vi "Window-Timelapse editor.vi"() -> ()   [LabVIEW 2013]
uses:
  User Interface/Visualisation/Timelapse Viewer/Typedefs/Custom slider-vertical.ctl
  User Interface/Visualisation/Timelapse Viewer/Typedefs/Timelapse viewer refs.ctl
  User Interface/Visualisation/Timelapse Viewer/Typedefs/Speed Viewer States enum.ctl
  <vilib>/Utility/miscctls.llb/LVPointTypeDef.ctl
  Typedefs/Save-Load enum.ctl
  <vilib>/vision/Image Controls.llb/IMAQ Image.ctl
  User Interface/Visualisation/Functional Imaging Viewer/Typedefs/Get-Set-Clear Control.ctl
  User Interface/Visualisation/Timelapse Viewer/Typedefs/Select Play-Stop button to show.ctl
  <vilib>/Utility/error.llb/DialogType.ctl
  User Interface/Visualisation/Timelapse Viewer/Cam video sync/Typedefs/Cam videos cluster.ctl
  User Interface/Visualisation/Timelapse Viewer/Globals/gl_Time series viewer globals.vi
  Global Variables/General Globals.vi
panel:
  out "Slider at frame #":i32 format="Slider at frame: %.0f"
  in  "Scrollbar":i32(c297)
  in  "Back":bool
  in  "Play":bool
  in  "Stop":bool
  in  "Tab Control":enum32{"Camera videos", "Speed data"}(tab)
  out "Cams":T2 {"Vid4 Rel time (ms)" format="%.0f ms"; "Vid3 Rel time (ms)" format="%.0f ms"; "Vid2 Rel time (ms)" format="%.0f ms"; "Vid1 Rel time (ms)" format="%.0f ms"}
  out "Actual number of speed points":i32 format="Actual of speed points: %.0f"
  out "Speed Data":string[][](array[string])
  out "Expected speed values":dbl format="Expected speed points: %#_g"
  out "Original frame rate (fps)":dbl format="Original frame rate: %#.1f (fps)"
  out "Frame rate set (fps)":dbl format="Frame rate set: %#.1f (fps)"
  out "Actual frame rate (fps)":dbl format="Actual frame rate: %#.1f (fps)"
  out "AVI Mode ind":string="AVI mode:"
  out "Video length info":string="Duration: 00h 00m 00s, 0 frames"
  in  "AVI File Path":path
  out "Export images":bool
  out "Export snippet":bool
  in  "Selection sliders":cluster{i32, i32}(slide)={1, 5594} scale=1.0..3919.0
  out "Export vid":bool
  out "Stop (ind)":bool
  in  "Intensity":T3={0.0, 4095.0} scale=0.0..4095.0
  in  "Colour":enum16{"Gray", "Red", "Green"}(ring)
  out "Speed Graph":dbl[](graph) caption="Speed Chart"
  out "Image":T1(plugin-control)
  # "Date                         Time                  Time stamp           Speed (rpm)          Angle (deg)"
  # "Time series info"
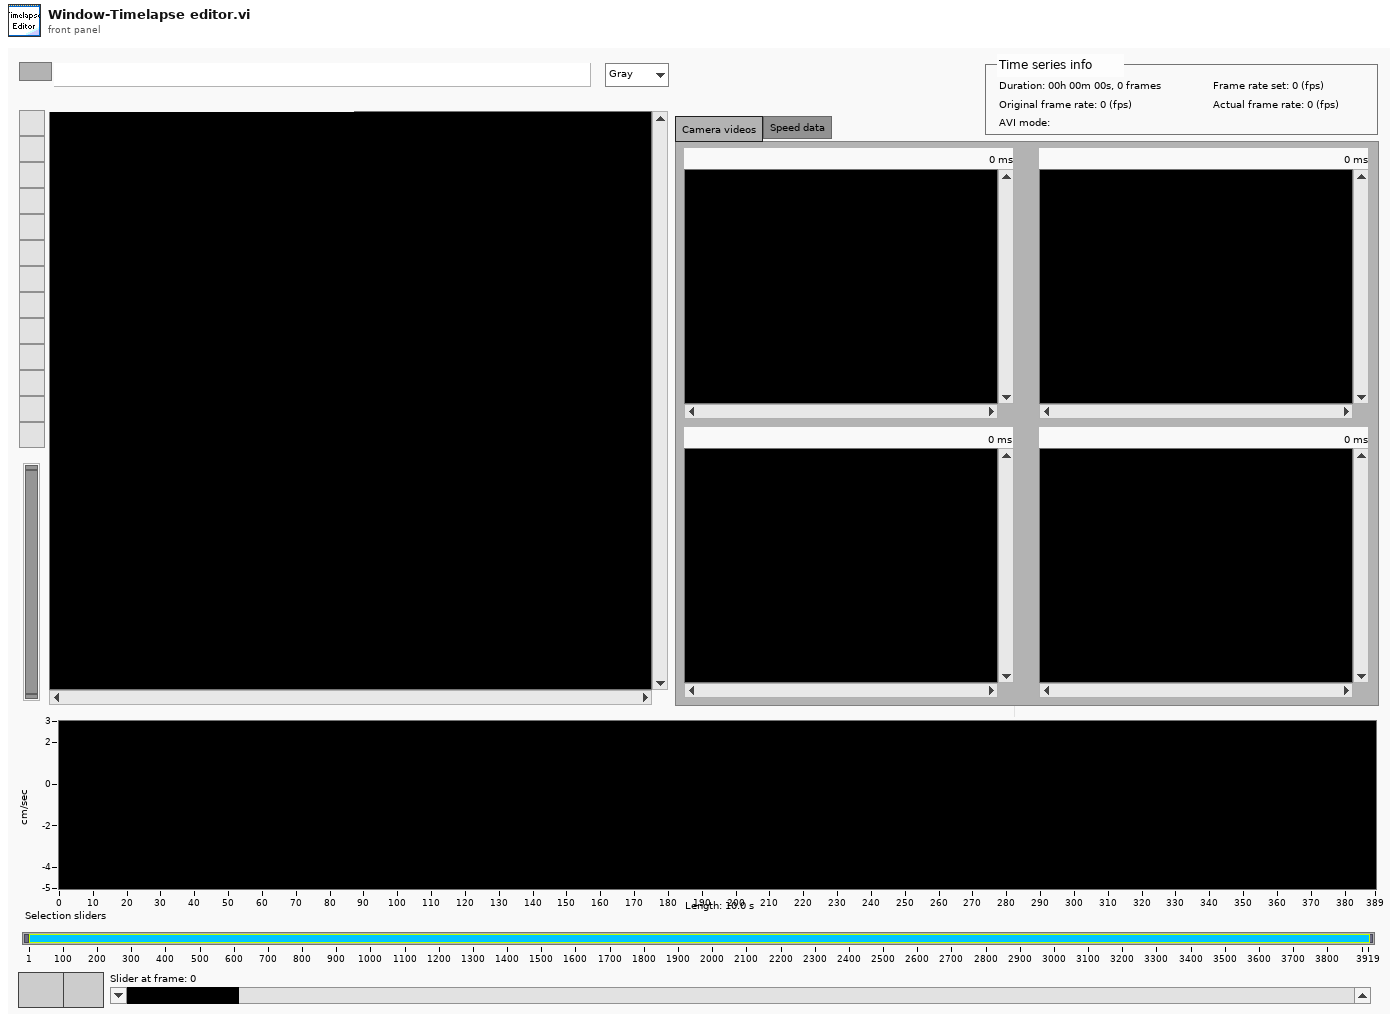
[diagram p1: front panel]
types:
  T1 = typedef "IMAQ Image.ctl" = refnum<image>
  T2 = cluster{"Vid 1":T1, "Vid 2":T1, "Vid 3":T1, "Vid 4":T1, "Vid1 Rel time (ms)":u32, "Vid2 Rel time (ms)":u32, "Vid3 Rel time (ms)":u32, "Vid4 Rel time (ms)":u32}
  T3 = typedef "Custom slider-vertical.ctl" = cluster{dbl, dbl}
  T4 = typedef "Timelapse viewer refs.ctl" = cluster{"This VI":refnum<vi>, "AVI Mode ind":refnum<vi>, "Play":refnum<vi>, "Stop":refnum<vi>, "Back":refnum<vi>, "Scrollbar":refnum<vi>, "Video length info":refnum<vi>, "Expected speed values":refnum<vi>, "Intensity":refnum<vi>, "Path":refnum<vi>, "Selection sliders":refnum<vi>, "Speed Graph ref":refnum<vi>, "Frame rate set (fps)":refnum<vi>}
  T5 = typedef "Save-Load enum.ctl" = enum16{"Save to file", "Load from file", "Compare from file"}
  T6 = enum16{"None", "Release queue", "Obtain queue", "Enqueue", "Get status", "Set status"}
  T7 = typedef "LVPointTypeDef.ctl" = cluster{"Horizontal":i16, "Vertical":i16}
  T8 = typedef "Speed Viewer States enum.ctl" = enum16{"Idle", "Initialise", "Playback", "Scroll bar event", "Speed cursor event", "Back to start", "Exit"}
  T9 = typedef "Image Type" = u32
  T10 = typedef "Custom slider-horisontal.ctl" = cluster{dbl, dbl}
  T11 = typedef "Get-Set-Clear Control.ctl" = enum16{"Get", "Set", "Clear"}
  T12 = typedef "Select Play-Stop button to show.ctl" = enum16{"Show Play button", "Show Stop button"}
  T13 = typedef "Cam videos cluster.ctl" = cluster{"Vid 1":T1, "Vid 2":T1, "Vid 3":T1, "Vid 4":T1, "Vid1 Rel time (ms)":u32, "Vid2 Rel time (ms)":u32, "Vid3 Rel time (ms)":u32, "Vid4 Rel time (ms)":u32}
  T14 = typedef "DialogType.ctl" = u16
  T15 = cluster{"Conversion Method":u32, "Minimum Value":i32, "Maximum Value":i32, "Number Of Shifts":i32}
  T16 = typedef "AVI modes refs cluster.ctl" = cluster{"AVI1 ref":T17, "AVI2 refs":T18[], "AVI # frames":u32[]}
  T17 = typedef "AviRefnum.ctl" = refnum<k1>
  T18 = typedef "IMAQ AVI2 Refnum.ctl" = refnum<k20>
  T19 = cluster{"Start Frame No":i32, "End Frame No":i32}
  T20 = typedef "AVI implementation enum.ctl" = enum16{"AVI1", "AVI2"}
  T21 = cluster{"# of frames to export":i32, "Initial frame's owning file":T18, "8-bit AVI file path":path, "Cursors location":cluster{"Number of first frame":i32, "Number of last frame":i32}}
  T22 = enum32{"Invalid", "Standard", "Closed", "Hidden", "Minimized", "Maximized"}
  T23 = typedef "Speed graph behaviour enum.ctl" = enum16{"Scrolling data", "Scrolling cursor"}
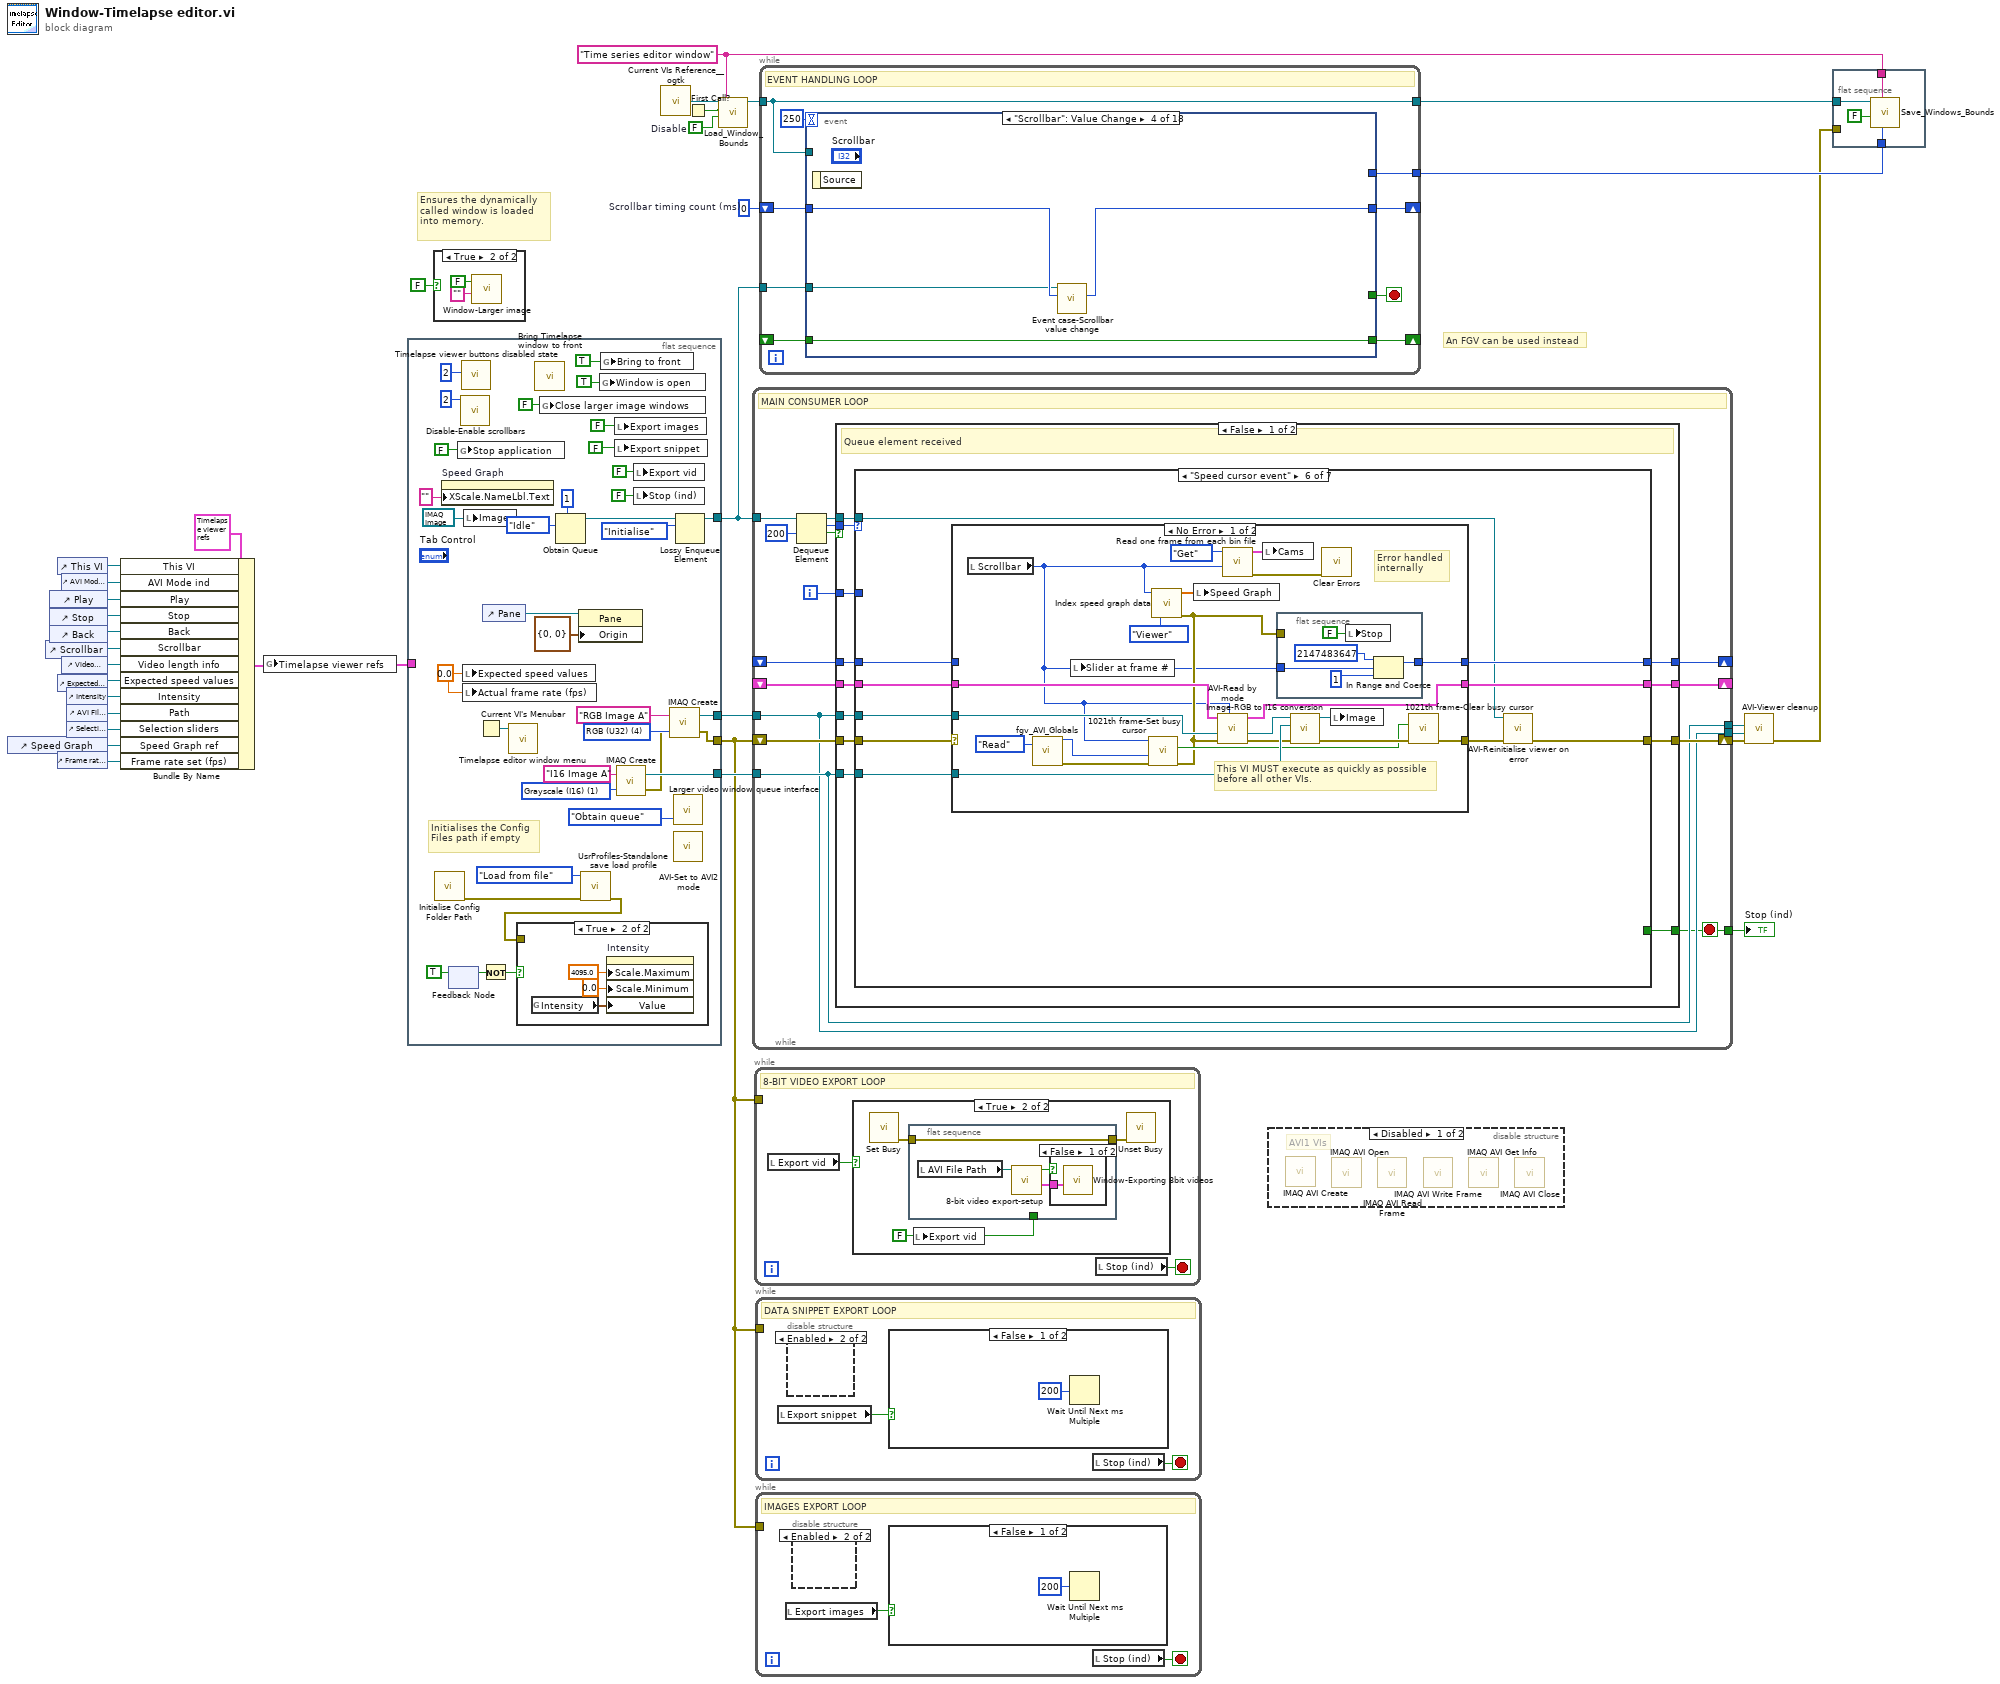
[diagram p0: block diagram]
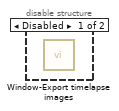
[diagram p3: hidden frame]
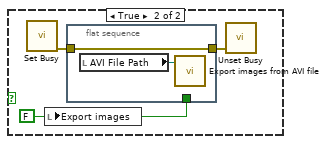
[diagram p4: hidden frame]
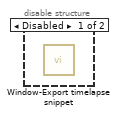
[diagram p5: hidden frame]
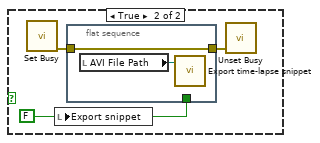
[diagram p6: hidden frame]
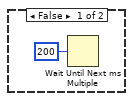
[diagram p8: hidden frame]
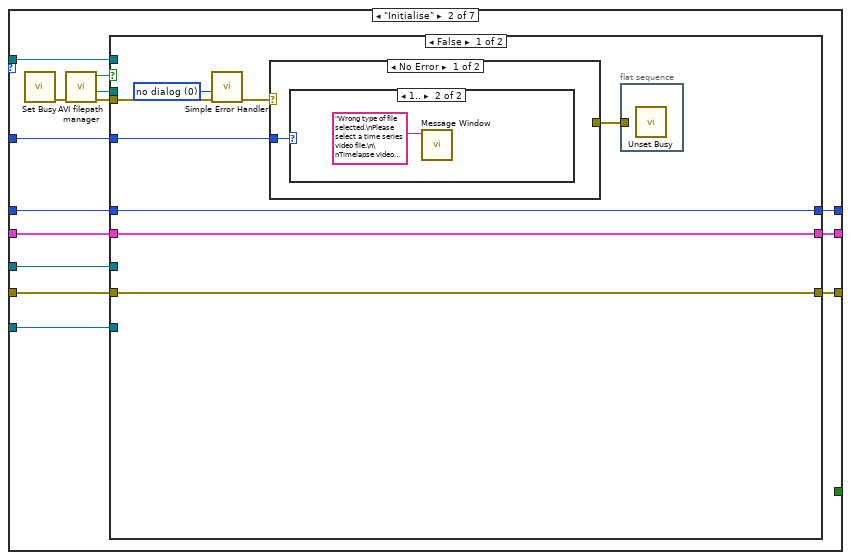
[diagram p12: hidden frame]
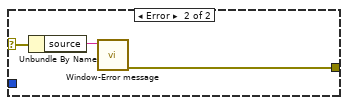
[diagram p14: hidden frame]
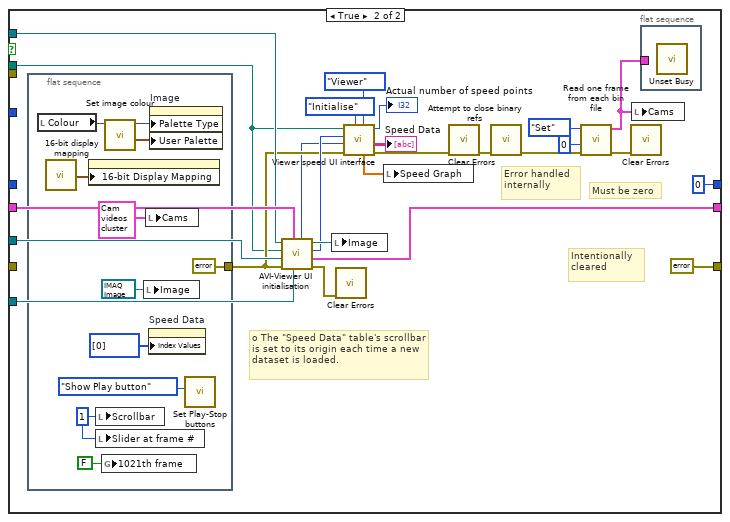
[diagram p15: hidden frame]
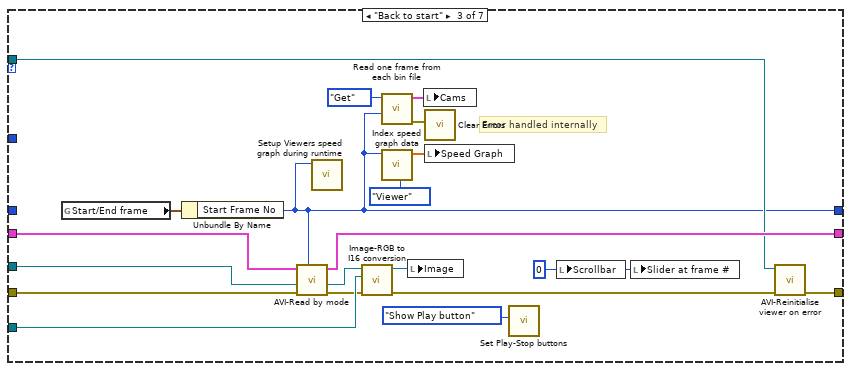
[diagram p16: hidden frame]
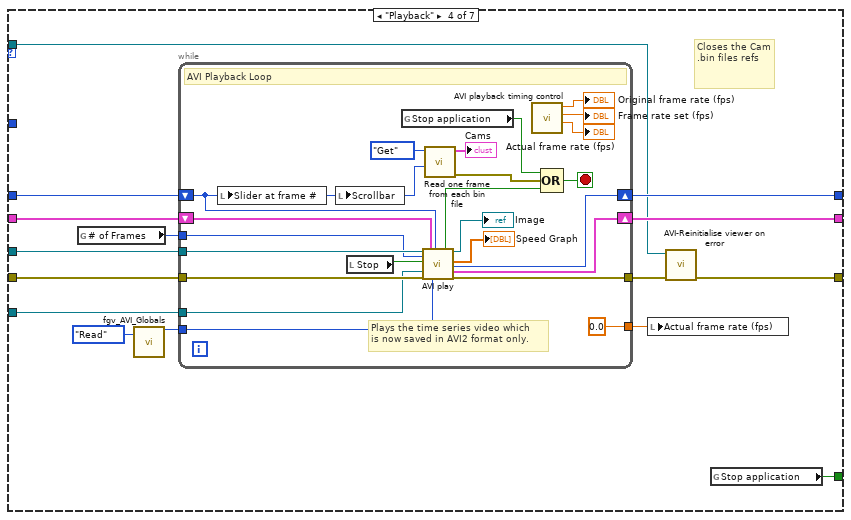
[diagram p17: hidden frame]
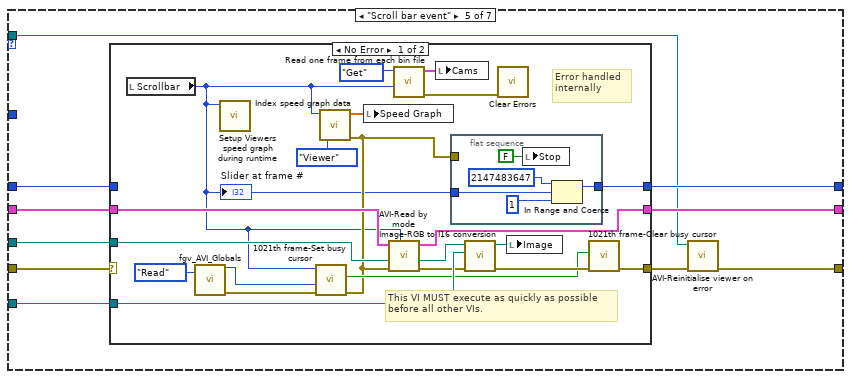
[diagram p18: hidden frame]
diagram:
  w8 = FALSE  # Disable
  w7 = "Time series editor window" ("Window Name (i.e. Key)")
  w19 = u32 0  # Scrollbar timing count (ms)
  # "Ensures the dynamically called window is loaded into memory."
  # "An FGV can be used instead"
  n1 = control-ref of="Speed Graph"() -> (w12:refnum<vi>)
  n2 = control-ref of="Scrollbar"() -> (w23:refnum<vi>)
  n3 = control-ref of="Play"() -> (w26:refnum<vi>)
  n4 = control-ref of="Stop"() -> (w25:refnum<vi>)
  n5 = control-ref of="Back"() -> (w24:refnum<vi>)
  n6 = control-ref of="This VI"() -> (w16:refnum<vi>)
  n7 = control-ref of="Expected speed values"() -> (w21:refnum<vi>)
  n8 = control-ref of="Frame rate set (fps)"() -> (w1:refnum<vi>)
  n9 = control-ref of="AVI Mode ind"() -> (w29:refnum<vi>)
  n10 = control-ref of="Video length info"() -> (w22:refnum<vi>)
  n11 = control-ref of="Intensity"() -> (w20:refnum<vi>)
  n12 = control-ref of="AVI File Path"() -> (w18:refnum<vi>)
  n13 = control-ref of="Selection sliders"() -> (w13:refnum<vi>)
  n14 = Bundle By Name(cluster=T4 {"This VI"=refnum, "AVI Mode ind"=refnum, "Play"=refnum, "Stop"=refnum, "Back"=refnum, "Scrollbar"=refnum, "Video length info"=refnum, "Expected speed values"=refnum, "Intensity"=refnum, "Path"=refnum, "Selection sliders"=refnum, "Speed Graph ref"=refnum, "Frame rate set (fps)"=refnum}, "This VI"=w16, "AVI Mode ind"=w29, "Play"=w26, "Stop"=w25, "Back"=w24, "Scrollbar"=w23, "Video length info"=w22, "Expected speed values"=w21, "Intensity"=w20, "Path"=w18, "Selection sliders"=w13, "Speed Graph ref"=w12, "Frame rate set (fps)"=w1) -> (w15:T4)
  n15 = global write "gl_Time series viewer globals.vi" "Timelapse viewer refs"(w15) -> ()
  n16 = flat-sequence {
    tunnel: [w67] -> w33
    tunnel: [w64] -> w32
    tunnel: [w57] -> w11
    tunnel: [w60] -> w30
    tunnel: w15 -> [_]
    frame #0 {
      w54 = 0.0 ("Expected speed points")
      w66 = T9 1 items=["Grayscale (U8)", "Grayscale (I16)", "Grayscale (SGL)", "Complex (CSG)", "RGB (U32)", "HSL (U32)", "RGB (U64)", "Grayscale (U16)"] ("Image Type")
      w68 = T9 4 items=["Grayscale (U8)", "Grayscale (I16)", "Grayscale (SGL)", "Complex (CSG)", "RGB (U32)", "HSL (U32)", "RGB (U64)", "Grayscale (U16)"] ("Image Type")
      # "Initialises the Config Files path if empty"
      n17 = call "Initialise Config Folder Path.vi"() -> ("error out"=w39:errorcluster)  [unwired: 9 in, 2 out]
      n18 = property on="Speed Graph" class="WFGraph (strict)"("XScale.NameLbl.Text"="" ("X Scale.Name Label.Text")) -> ()  [unwired: 2 in, 2 out]
      n19 = feedback #1() -> (w34:bool)  [unwired: 1 in]
      n20 = feedback-in #1(TRUE) -> ()
      n21 = global write "General Globals.vi" "Stop application"(FALSE ("Stop application")) -> ()
      n22 = call "Disable-Enable scrollbars.vi"("Disabled state"=2) -> ()  [unwired: 10 in, 1 out]
      n23 = call "Timelapse viewer buttons disabled state.vi"("Disabled"=2) -> ()  [unwired: 10 in, 1 out]
      n24 = local write "Expected speed values"(w54) -> ()
      n25 = local write "Actual frame rate (fps)"(w54) -> ()
      n26 = local write "Image"(T1 refnum ("Image")) -> ()
      n27 = Current VI's Menubar() -> (w53:refnum<k9>)
      n28 = Not(x=w34) -> (.not. x?=w37:bool)
      n29 = control-ref of="Pane"() -> (w55:refnum<vi>)
      n30 = call "Timelapse editor window menu.vi"("menu"=w53) -> ()  [unwired: 9 in, 2 out]
      n31 = call "Bring Timelapse window to front.vi"() -> ()  [unwired: 12 in]
      n32 = global write "gl_Time series viewer globals.vi" "Close larger image windows"(FALSE ("Close larger image window")) -> ()
      n33 = Obtain Queue(max queue size (-1, unlimited)=1, element data type=Speed_Viewer_States_enum."Idle" ("States")) -> (queue out=w61:refnum<queue>)  [unwired: 3 in, 2 out]
      n34 = property class="Pane"(reference=w55, "Origin"=T7 {"Horizontal"=0, "Vertical"=0}) -> ()  [unwired: 1 in, 2 out]
      n35 = call "UsrProfiles-Standalone save load profile.vi"("Error in"=w39, "Function"=Save-Load_enum."Load from file") -> ("error out"=w36:errorcluster)  [unwired: 9 in]
      n36 = case shown="True" w37 {
        tunnel: w36 -> [_ _]
        frame False {
        }
        frame True {
          n37 = global read "gl_Time series viewer globals.vi" "Intensity"() -> (w70:T10)
          n38 = property on="Intensity" class="Slide (strict)"("Scale.Maximum"=4095.0 ("Scale.Range:Maximum"), "Scale.Minimum"=0.0 ("Scale.Range:Minimum"), "Value"=w70) -> ()  [unwired: 2 in, 2 out]
        }
      }
      n39 = global write "gl_Time series viewer globals.vi" "Window is open"(TRUE ("Window is open")) -> ()
      n40 = global write "gl_Time series viewer globals.vi" "Bring to front"(TRUE ("Bring Timelapse Editor to front")) -> ()
      n41 = local write "Export images"(FALSE ("Export data subset")) -> ()
      n42 = local write "Export snippet"(FALSE ("Export data subset")) -> ()
      n43 = call "IMAQ Create"("Image Name"="I16 Image A", "Image Type"=w66) -> ("New Image"=w64:T1, "error out"=w58:errorcluster)  [unwired: 2 in, 1 out]
      n44 = local write "Export vid"(FALSE ("Export")) -> ()
      n45 = local write "Stop (ind)"(FALSE ("Boolean")) -> ()
      n46 = call "IMAQ Create"("Image Name"="RGB Image A", "Image Type"=w68, "error in (no error)"=w58) -> ("New Image"=w67:T1, "error out"=w57:errorcluster)  [unwired: 1 in, 1 out]
      n47 = call "Larger video window queue interface.vi"("Function"=T6."Obtain queue") -> ()  [unwired: 10 in, 1 out]
      n48 = call "AVI-Set to AVI2 mode.vi"() -> ()  [unwired: 11 in, 1 out]
      n49 = Lossy Enqueue Element(queue=w61, element=Speed_Viewer_States_enum."Initialise" ("States")) -> (queue out=w60:refnum<queue>)  [unwired: 1 in, 3 out]
    }
  }
  n50 = case shown="True" FALSE {
    frame False {
    }
    frame True {
      n51 = call "Window-Larger image.vi"("Image name"="", "Open maximised"=FALSE) -> ()  [unwired: 10 in]
    }
  }
  n52 = call "Current VIs Reference__ogtk.vi"() -> ("Current VI's reference"=w10:refnum<vi>)  [unwired: 5 in]
  n53 = First Call?() -> (First Call?: T/F=w9:bool)
  n54 = call "Load_Window_Bounds.vi"("Window Name (i.e. Key)"=w7, "Disable"=w8, "First Call"=w9, "Window VI's Ref"=w10) -> ("reference out"=w4:refnum<vi>)  [unwired: 4 in, 3 out]
  n55 = while {
    tunnel: w33 -> [w78]
    tunnel: w32 -> [w79]
    tunnel: [w79] -> w31
    shift-right: [w86] -> _
    shift-left: _ -> [w85]
    tunnel: w30 -> [w84]
    shift-right: [w80] -> _
    shift-left: _ -> [w89]
    tunnel: [w78] -> w17
    shift-right: [w87] -> w27
    shift-left: w11 -> [w88]
    tunnel: [w76] -> w14
    i -> [w75]
    stop <- w76 stop-if-true
    # "MAIN CONSUMER LOOP"
    n56 = Dequeue Element(queue=w84, timeout in ms (-1)=200) -> (queue out=w77:refnum<queue>, element=w81:T8, timed out?=w82:bool)  [unwired: 1 in, 1 out]
    n57 = case shown="False" w82 {
      tunnel: w89 -> [w101 w314]
      tunnel: [w100 w314] -> w80
      tunnel: w78 -> [w99 _]
      tunnel: w79 -> [w98 _]
      tunnel: w88 -> [w97 w313]
      tunnel: [w96 w313] -> w87
      tunnel: [w95 w315] -> w86
      tunnel: w85 -> [w94 w315]
      tunnel: w81 -> [w93 _]
      tunnel: [w92 w312] -> w76
      tunnel: w77 -> [w91 _]
      tunnel: w75 -> [w90 _]
      frame False {
        # "Queue element received"
        n58 = case shown="\"Speed cursor event\"" w93 {
          tunnel: w101 -> [w103 w118 w185 w202 w231 w270 w306]
          tunnel: [w103 w114 w184 w196 w233 w272 w306] -> w100
          tunnel: w99 -> [_ w113 w182 w201 w232 w271 _]
          tunnel: w98 -> [_ w112 w183 w200 w235 w274 _]
          tunnel: w97 -> [w102 w116 w180 w199 w230 w269 w305]
          tunnel: [w102 w115 w175 w195 w228 w267 w304] -> w96
          tunnel: [w104 w117 w168 w198 w234 w273 1 ("Slide")] -> w95
          tunnel: w94 -> [w104 w111 _ w197 w229 w268 _]
          tunnel: [_ _ _ w188 _ _ TRUE] -> w92
          tunnel: w91 -> [_ w107 w174 w193 w226 w265 _]
          tunnel: w90 -> [_ w106 _ _ _ _ _]
          frame Default {
          }
          frame "Initialise" {
            n59 = call <vilib>:"Set Busy.vi"() -> ("error out"=w105:errorcluster)  [unwired: 10 in, 1 out]
            n60 = call "AVI filepath manager.vi"("error in (no error)"=w105) -> ("error"=w108:errorcluster, "AVI File Path"=w109:path, "File path OK"=w110:bool)  [unwired: 8 in]
            n61 = case shown="False" w110 {
              tunnel: w118 -> [w125 w156]
              tunnel: [w126 0 ("Slide")] -> w117
              tunnel: w109 -> [_ w140]
              tunnel: w116 -> [w124 _]
              tunnel: [w124 errorcluster {"status"=FALSE, "code"=0, "source"=""} ("error out")] -> w115
              tunnel: [w125 w149] -> w114
              tunnel: w113 -> [_ w148]
              tunnel: w112 -> [_ w154]
              tunnel: w111 -> [w126 _]
              tunnel: w108 -> [w123 _]
              tunnel: w107 -> [_ w152]
              tunnel: w106 -> [w120 _]
              frame False {
                w122 = T14 0 items=["no dialog", "OK message", "continue or stop message", "OK message + warnings", "continue/stop + warnings"] ("type of dialog (OK msg:1)")
                n62 = call <vilib>:"Simple Error Handler.vi"("type of dialog (OK msg:1)"=w122, "error in (no error)"=w123) -> ("error out"=w121:errorcluster)  [unwired: 3 in, 4 out]
                n63 = case shown="No Error" w121 {
                  selector: w121 -> [_ w131]
                  tunnel: w120 -> [w127 _]
                  tunnel: [_ w129] -> w119
                  frame No Error {
                    n64 = case shown="1.." w127 {
                      frame 0, Default {
                      }
                      frame 1.. {
                        n65 = call "Message Window.vi"("Message string"="Wrong type of file selected.\nPlease select a time series video file.\n\nTimelapse video files are located  in time series folders \ne.g. \"TimeLapse 02_10_2014 20-22-02\"\nand their file names are similar to this: \"Green Channel 1\"\n\nNote: For time series video files which are part of a split-files sequence e.g. Green Channel 1, Green Channel 2, Green Channel 3... \ndouble click on any one file. The full sequence will open in the viewer regardless of which file you select.") -> ()  [unwired: 10 in, 1 out]
                      }
                    }
                  }
                  frame Error {
                    n66 = Unbundle By Name(w131) -> ("source"=w130:string)
                    n67 = call "Window-Error message.vi"("Message"=w130) -> ("Error Out (no error)"=w129:errorcluster)  [unwired: 10 in]
                  }
                }
                n68 = flat-sequence {
                  tunnel: w119 -> [_]
                  frame #0 {
                    n69 = call <vilib>:"Unset Busy.vi"() -> ()  [unwired: 11 in, 1 out]
                  }
                }
              }
              frame True {
                # "Must be zero"
                # "o\tThe \"Speed Data\" table's scrollbar is set to its origin each time a new dataset is loaded."
                # "Error handled internally"
                # "Intentionally cleared"
                n70 = flat-sequence {
                  tunnel: [errorcluster {"status"=FALSE, "code"=0, "source"=""} ("error out")] -> w141
                  frame #0 {
                    w158 = 1 ("Scrollbar")
                    n71 = local read "Colour"() -> (w164:enum16{"Gray", "Red", "Green"})
                    n72 = call "16-bit display mapping.vi"() -> ("16-bit Display Mapping"=w161:T15)  [unwired: 10 in, 1 out]
                    n73 = property on="Image" class="ImageControl"("16-bit Display Mapping"=w161) -> ()  [unwired: 2 in, 2 out]
                    n74 = local write "Scrollbar"(w158) -> ()
                    n75 = local write "Slider at frame #"(w158) -> ()
                    n76 = global write "gl_Time series viewer globals.vi" "1021th frame"(FALSE ("1021th frame")) -> ()
                    n77 = call "Set image colour.vi"("Left Image Palette"=w164) -> ("Color Palette"=w162:cluster{"Red":u8, "Green":u8, "Blue":u8}[], "Palette Type"=w163:u32)  [unwired: 9 in]
                    n78 = local write "Image"(T1 refnum ("New Image")) -> ()
                    n79 = local write "Cams"(T13 {"Vid 1"=refnum, "Vid 2"=refnum, "Vid 3"=refnum, "Vid 4"=refnum, "Vid1 Rel time (ms)"=0, "Vid2 Rel time (ms)"=0, "Vid3 Rel time (ms)"=0, "Vid4 Rel time (ms)"=0} ("Cam videos cluster")) -> ()
                    n80 = property on="Speed Data" class="Arr (strict)"("Index Values"=u32[] [0]) -> ()  [unwired: 2 in, 2 out]
                    n81 = property on="Image" class="ImageControl"("Palette Type"=w163, "User Palette"=w162) -> ()  [unwired: 2 in, 2 out]
                    n82 = call "Set Play-Stop buttons.vi"("Function"=Select_Play-Stop_button_to_show."Show Play button") -> ()  [unwired: 10 in, 1 out]
                  }
                }
                n83 = call "AVI-Viewer UI initialisation.vi"("I16 image ref in"=w154, "AVI modes refs in"=w156, "error in (no error)"=w141, "RGB image ref in"=w148, "AVI File Path"=w140, "Queue in"=w152) -> ("error out"=w135:errorcluster, "AVI modes refs out"=w149:T16, "Number of Frames"=w150:u32, "Refnum out"=w151:T1, "Scrollbar position"=w134:i32)  [unwired: 1 in]
                n84 = local write "Image"(w151) -> ()
                n85 = call <vilib>:"Clear Errors.vi"("error in (no error)"=w135) -> ()  [unwired: 6 in, 1 out]
                n86 = call "Viewer speed UI interface.vi"("Caller"=enum16{"Viewer", "Exporter"}."Viewer", "Function"=enum16{"Initialise", "Update"}."Initialise", "error in (no error)"=w141, "Gobal frame number in Timelapse data/master video (1 based)"=w134, "Number of Frames"=w150, "Speed Data folder path+dummy filename"=w140) -> ("error out"=w146:errorcluster, "Speed Data"=→"Speed Data":string[][], "Actual number of speed values"=→"Actual number of speed points":i32, "Speed waveform graph data"=w155:dbl[])  [unwired: 2 in]
                n87 = local write "Speed Graph"(w155) -> ()
                n88 = call <vilib>:"Clear Errors.vi"("error in (no error)"=w146) -> ("error out"=w142:errorcluster)  [unwired: 6 in]
                n89 = call "Attempt to close binary refs.vi"("error in (no error)"=w142) -> ("error out"=w143:errorcluster)  [unwired: 10 in]
                n90 = call "Read one frame from each bin file.vi"("error in (no error)"=w143, "Master video's frame number (unity-based)"=0 ("Frame number"), "Get/set"=Get-Set-Clear_Control."Set" ("GEt set .bin refs")) -> ("Error out"=w136:errorcluster, "Cam videos cluster"=w139:T13)  [unwired: 7 in]
                n91 = call <vilib>:"Clear Errors.vi"("error in (no error)"=w136) -> ()  [unwired: 6 in, 1 out]
                n92 = local write "Cams"(w139) -> ()
                n93 = flat-sequence {
                  tunnel: w139 -> [_]
                  frame #0 {
                    n94 = call <vilib>:"Unset Busy.vi"() -> ()  [unwired: 11 in, 1 out]
                  }
                }
              }
            }
          }
          frame "Back to start" {
            w187 = 0 ("Scrollbar")
            # "Error handled internally"
            n95 = global read "gl_Time series viewer globals.vi" "Start/End frame"() -> (w169:T19)
            n96 = Unbundle By Name(w169) -> ("Start Frame No"=w168:i32)
            n97 = call "AVI-Read by mode.vi"("Frame number (unity-based)"=w168, "error in (no error)"=w180, "RGB image ref in"=w182, "AVI modes refs"=w185) -> ("error out"=w179:errorcluster, "RGB image ref out"=w186:T1, "AVI modes refs"=w184:T16)  [unwired: 5 in]
            n98 = call "Setup Viewers speed graph during runtime.vi"("Frame number"=w168) -> ()  [unwired: 10 in, 1 out]
            n99 = call "Image-RGB to I16 conversion.vi"("error in (no error)"=w179, "I16 image ref in"=w183, "RGB image ref in"=w186) -> ("error out"=w176:errorcluster, "I16 image ref out"=w181:T1)  [unwired: 7 in]
            n100 = call "Read one frame from each bin file.vi"("Master video's frame number (unity-based)"=w168, "Get/set"=Get-Set-Clear_Control."Get" ("GEt set .bin refs")) -> ("Error out"=w171:errorcluster, "Cam videos cluster"=w173:T13)  [unwired: 8 in]
            n101 = call "Index speed graph data.vi"("Caller"=enum16{"Viewer", "Exporter"}."Viewer", "Gobal frame number in Timelapse data/master video (1 based)"=w168) -> ("Speed data waveform graph"=w177:dbl[])  [unwired: 7 in, 2 out]
            n102 = local write "Image"(w181) -> ()
            n103 = local write "Cams"(w173) -> ()
            n104 = call <vilib>:"Clear Errors.vi"("error in (no error)"=w171) -> ()  [unwired: 6 in, 1 out]
            n105 = local write "Speed Graph"(w177) -> ()
            n106 = call "Set Play-Stop buttons.vi"("Function"=Select_Play-Stop_button_to_show."Show Play button") -> ()  [unwired: 10 in, 1 out]
            n107 = local write "Scrollbar"(w187) -> ()
            n108 = local write "Slider at frame #"(w187) -> ()
            n109 = call "AVI-Reinitialise viewer on error.vi"("error in (no error)"=w176, "Queue in"=w174) -> ("error out"=w175:errorcluster)  [unwired: 9 in]
          }
          frame "Playback" {
            # "Closes the Cam .bin files refs"
            n110 = global read "gl_Time series viewer globals.vi" "# of Frames"() -> (w190:u32)
            n111 = call "fgv_AVI_Globals.vi"("Function"=enum16{"Intialize", "Write", "Read", "Clear"}."Read") -> ("AVI mode"=w191:T20)  [unwired: 11 in, 3 out]
            n112 = while {
              tunnel: w201 -> [w223]
              tunnel: w200 -> [w213]
              tunnel: w199 -> [w221]
              tunnel: [w222] -> w194
              shift-right: [w219] -> w198
              shift-left: w197 -> [w208]
              shift-right: [w224] -> w196
              shift-left: w202 -> [w225]
              tunnel: w191 -> [w215]
              tunnel: w190 -> [w212]
              tunnel: [0.0 ("Expected speed points")] -> w189
              stop <- w205 stop-if-true
              # "Plays the time series video which \nis now saved in AVI2 format only."
              # "AVI Playback Loop"
              n113 = local write "Slider at frame #"(w208) -> ()
              n114 = local write "Scrollbar"(w208) -> ()
              n115 = local read "Stop"() -> (w214:bool)
              n116 = global read "General Globals.vi" "Stop application"() -> (w203:bool)
              n117 = call "AVI play.vi"("RGB Image ref"=w223, "Number of Frames"=w212, "Stop button pressed"=w214, "I16 Image ref"=w213, "error in (no error)"=w221, "AVI modes refs in"=w225, "AVI mode"=w215, "Frame number (in)"=w208) -> ("Playback stopped"=w206:bool, "I16 image ref out"=→"Image":T1, "Speed data waveform graph"=→"Speed Graph":dbl[], "Frame number (out)"=w219:i32, "AVI modes refs out"=w224:T16, "error out"=w222:errorcluster)  [unwired: 6 in]
              n118 = call "Read one frame from each bin file.vi"("Master video's frame number (unity-based)"=w208, "Get/set"=Get-Set-Clear_Control."Get" ("GEt set .bin refs")) -> ("Error out"=w204:errorcluster, "Cam videos cluster"=→"Cams":T13)  [unwired: 8 in]
              n119 = call "AVI playback timing control.vi"() -> ("Actual frame rate (fps)"=→"Actual frame rate (fps)":dbl, "Frame rate set OR original (fps)"=→"Frame rate set (fps)":dbl, "Original frame rate (fps)"=→"Original frame rate (fps)":dbl)  [unwired: 8 in, 1 out]
              n120 = Compound Arithmetic op=OR(w203, w204, w206) -> (w205:bool)
            }
            n121 = local write "Actual frame rate (fps)"(w189) -> ()
            n122 = call "AVI-Reinitialise viewer on error.vi"("error in (no error)"=w194, "Queue in"=w193) -> ("error out"=w195:errorcluster)  [unwired: 9 in]
            n123 = global read "General Globals.vi" "Stop application"() -> (w188:bool)
          }
          frame "Scroll bar event" {
            n124 = case shown="No Error" w230 {
              selector: w230 -> [_ w264]
              tunnel: w235 -> [w256 _]
              tunnel: [w254 w263] -> w234
              tunnel: [w243 w262] -> w233
              tunnel: w232 -> [w252 _]
              tunnel: w231 -> [w250 w262]
              tunnel: [w245 w264] -> w227
              tunnel: w229 -> [_ w263]
              frame No Error {
                # "Error handled internally"
                # "This VI MUST execute as quickly as possible\nbefore all other VIs."
                n125 = local read "Scrollbar"() -> (w236:i32)
                "Slider at frame #" <- w236
                n126 = call "fgv_AVI_Globals.vi"("Function"=enum16{"Intialize", "Write", "Read", "Clear"}."Read") -> ("AVI mode"=w248:T20, "error out"=w247:errorcluster)  [unwired: 11 in, 2 out]
                n127 = call "Setup Viewers speed graph during runtime.vi"("Frame number"=w236) -> ()  [unwired: 10 in, 1 out]
                n128 = call "1021th frame-Set busy cursor.vi"("error in (no error)"=w247, "AVI mode"=w248, "Frame number"=w236) -> ("error out"=w238:errorcluster, "Busy cursor was set"=w244:bool)  [unwired: 7 in]
                n129 = call "Index speed graph data.vi"("Caller"=enum16{"Viewer", "Exporter"}."Viewer", "error in (no error)"=w238, "Gobal frame number in Timelapse data/master video (1 based)"=w236) -> ("Speed data waveform graph"=w239:dbl[])  [unwired: 6 in, 2 out]
                n130 = local write "Speed Graph"(w239) -> ()
                n131 = call "AVI-Read by mode.vi"("Frame number (unity-based)"=w236, "error in (no error)"=w238, "RGB image ref in"=w252, "AVI modes refs"=w250) -> ("error out"=w253:errorcluster, "RGB image ref out"=w251:T1, "AVI modes refs"=w243:T16)  [unwired: 5 in]
                n132 = call "Read one frame from each bin file.vi"("Master video's frame number (unity-based)"=w236, "Get/set"=Get-Set-Clear_Control."Get" ("GEt set .bin refs")) -> ("Error out"=w240:errorcluster, "Cam videos cluster"=w242:T13)  [unwired: 8 in]
                n133 = local write "Cams"(w242) -> ()
                n134 = flat-sequence {
                  tunnel: [w259] -> w254
                  tunnel: w236 -> [w257]
                  tunnel: w238 -> [_]
                  frame #0 {
                    n135 = local write "Stop"(FALSE ("Stop")) -> ()
                    n136 = In Range and Coerce(upper limit=2147483647, x=w257, lower limit=1) -> (coerced(x)=w259:i32)  [unwired: 1 out]
                  }
                }
                n137 = call "Image-RGB to I16 conversion.vi"("error in (no error)"=w253, "I16 image ref in"=w256, "RGB image ref in"=w251) -> ("error out"=w246:errorcluster, "I16 image ref out"=w255:T1)  [unwired: 7 in]
                n138 = call <vilib>:"Clear Errors.vi"("error in (no error)"=w240) -> ()  [unwired: 6 in, 1 out]
                n139 = local write "Image"(w255) -> ()
                n140 = call "1021th frame-Clear busy cursor.vi"("error in (no error)"=w246, "Busy cursor was set"=w244) -> ("error out"=w245:errorcluster)  [unwired: 9 in]
              }
              frame Error {
              }
            }
            n141 = call "AVI-Reinitialise viewer on error.vi"("error in (no error)"=w227, "Queue in"=w226) -> ("error out"=w228:errorcluster)  [unwired: 9 in]
          }
          frame "Speed cursor event" {
            n142 = case shown="No Error" w269 {
              selector: w269 -> [_ w303]
              tunnel: w274 -> [w295 _]
              tunnel: [w293 w302] -> w273
              tunnel: [w282 w301] -> w272
              tunnel: w271 -> [w291 _]
              tunnel: w270 -> [w289 w301]
              tunnel: [w284 w303] -> w266
              tunnel: w268 -> [_ w302]
              frame No Error {
                # "Error handled internally"
                # "This VI MUST execute as quickly as possible\nbefore all other VIs."
                n143 = local read "Scrollbar"() -> (w275:i32)
                n144 = call "fgv_AVI_Globals.vi"("Function"=enum16{"Intialize", "Write", "Read", "Clear"}."Read") -> ("AVI mode"=w287:T20, "error out"=w286:errorcluster)  [unwired: 11 in, 2 out]
                n145 = local write "Slider at frame #"(w275) -> ()
                n146 = call "1021th frame-Set busy cursor.vi"("error in (no error)"=w286, "AVI mode"=w287, "Frame number"=w275) -> ("error out"=w277:errorcluster, "Busy cursor was set"=w283:bool)  [unwired: 7 in]
                n147 = call "Index speed graph data.vi"("Caller"=enum16{"Viewer", "Exporter"}."Viewer", "error in (no error)"=w277, "Gobal frame number in Timelapse data/master video (1 based)"=w275) -> ("Speed data waveform graph"=w278:dbl[])  [unwired: 6 in, 2 out]
                n148 = local write "Speed Graph"(w278) -> ()
                n149 = call "AVI-Read by mode.vi"("Frame number (unity-based)"=w275, "error in (no error)"=w277, "RGB image ref in"=w291, "AVI modes refs"=w289) -> ("error out"=w292:errorcluster, "RGB image ref out"=w290:T1, "AVI modes refs"=w282:T16)  [unwired: 5 in]
                n150 = call "Read one frame from each bin file.vi"("Master video's frame number (unity-based)"=w275, "Get/set"=Get-Set-Clear_Control."Get" ("GEt set .bin refs")) -> ("Error out"=w279:errorcluster, "Cam videos cluster"=w281:T13)  [unwired: 8 in]
                n151 = local write "Cams"(w281) -> ()
                n152 = flat-sequence {
                  tunnel: [w298] -> w293
                  tunnel: w275 -> [w296]
                  tunnel: w277 -> [_]
                  frame #0 {
                    n153 = local write "Stop"(FALSE ("Stop")) -> ()
                    n154 = In Range and Coerce(upper limit=2147483647, x=w296, lower limit=1) -> (coerced(x)=w298:i32)  [unwired: 1 out]
                  }
                }
                n155 = call "Image-RGB to I16 conversion.vi"("error in (no error)"=w292, "I16 image ref in"=w295, "RGB image ref in"=w290) -> ("error out"=w285:errorcluster, "I16 image ref out"=w294:T1)  [unwired: 7 in]
                n156 = call <vilib>:"Clear Errors.vi"("error in (no error)"=w279) -> ()  [unwired: 6 in, 1 out]
                n157 = local write "Image"(w294) -> ()
                n158 = call "1021th frame-Clear busy cursor.vi"("error in (no error)"=w285, "Busy cursor was set"=w283) -> ("error out"=w284:errorcluster)  [unwired: 9 in]
              }
              frame Error {
              }
            }
            n159 = call "AVI-Reinitialise viewer on error.vi"("error in (no error)"=w266, "Queue in"=w265) -> ("error out"=w267:errorcluster)  [unwired: 9 in]
          }
          frame "Exit" {
            n160 = local read "Stop"() -> (w310:bool)
            n161 = Unbundle By Name(w306) -> ("AVI2 refs"=w307:T18[])
            n162 = case shown="True" w310 {
              frame False {
              }
              frame True {
                n163 = local write "Stop"(FALSE ("Stop")) -> ()
              }
            }
            n164 = call "AVI-AVI2 Close all.vi"("error in (no error)"=w305, "AVI2 ref"=w307) -> ("error out"=w304:errorcluster)  [unwired: 9 in]
          }
        }
      }
      frame True {
        # "Timeout"
        n165 = global read "General Globals.vi" "Stop application"() -> (w312:bool)
      }
    }
  }
  "Stop (ind)" <- w14
  n166 = while {
    tunnel: w11 -> [_]
    stop <- w317 stop-if-true
    # "8-BIT VIDEO EXPORT LOOP"
    n167 = local read "Export vid"() -> (w316:bool)
    n168 = case shown="True" w316 {
      frame False {
        n169 = Wait Until Next ms Multiple(millisecond multiple=u32 200) -> ()  [unwired: 1 out]
      }
      frame True {
        w321 = FALSE ("Export")
        n170 = call <vilib>:"Set Busy.vi"() -> ("error out"=w320:errorcluster)  [unwired: 10 in, 1 out]
        n171 = flat-sequence {
          tunnel: w321 -> [_]
          tunnel: w320 -> [w325]
          tunnel: [w325] -> w319
          frame #0 {
            n172 = local read "AVI File Path"() -> (w324:path)
            n173 = call "8-bit video export-setup.vi"("selected AVI file path"=w324) -> ("output cluster"=w323:T21, "cancelled"=w322:bool)  [unwired: 9 in]
            n174 = case shown="False" w322 {
              tunnel: w323 -> [w326 _]
              frame False {
                n175 = call "Window-Exporting 8bit videos.vi"("Input cluster"=w326) -> ()  [unwired: 11 in]
              }
              frame True {
              }
            }
          }
        }
        n176 = local write "Export vid"(w321) -> ()
        n177 = call <vilib>:"Unset Busy.vi"("error in (no error)"=w319) -> ()  [unwired: 10 in, 1 out]
      }
    }
    n178 = local read "Stop (ind)"() -> (w317:bool)
  }
  n179 = while {
    tunnel: w11 -> [_]
    stop <- w328 stop-if-true
    # "DATA SNIPPET EXPORT LOOP"
    n180 = local read "Export snippet"() -> (w327:bool)
    n181 = disable-structure shown="Enabled" {
      frame Disabled {
        n182 = call "Window-Export timelapse snippet.vi"() -> ()  [unwired: 12 in]
      }
      frame Enabled {
      }
    }
    n183 = case shown="False" w327 {
      frame False {
        n184 = Wait Until Next ms Multiple(millisecond multiple=u32 200) -> ()  [unwired: 1 out]
      }
      frame True {
        w332 = FALSE ("Export data subset")
        n185 = call <vilib>:"Set Busy.vi"() -> ("error out"=w331:errorcluster)  [unwired: 10 in, 1 out]
        n186 = local write "Export snippet"(w332) -> ()
        n187 = flat-sequence {
          tunnel: w332 -> [_]
          tunnel: w331 -> [w334]
          tunnel: [w334] -> w330
          frame #0 {
            n188 = local read "AVI File Path"() -> (w333:path)
            n189 = call "Export time-lapse snippet.vi"("AVI File Path"=w333) -> ()  [unwired: 11 in]
          }
        }
        n190 = call <vilib>:"Unset Busy.vi"("error in (no error)"=w330) -> ()  [unwired: 10 in, 1 out]
      }
    }
    n191 = local read "Stop (ind)"() -> (w328:bool)
  }
  n192 = while {
    tunnel: w11 -> [_]
    stop <- w336 stop-if-true
    # "IMAGES EXPORT LOOP"
    n193 = local read "Export images"() -> (w335:bool)
    n194 = disable-structure shown="Enabled" {
      frame Disabled {
        n195 = call "Window-Export timelapse images.vi"() -> ()  [unwired: 12 in]
      }
      frame Enabled {
      }
    }
    n196 = case shown="False" w335 {
      frame False {
        n197 = Wait Until Next ms Multiple(millisecond multiple=u32 200) -> ()  [unwired: 1 out]
      }
      frame True {
        w338 = FALSE ("Export data subset")
        n198 = call <vilib>:"Set Busy.vi"() -> ("error out"=w340:errorcluster)  [unwired: 10 in, 1 out]
        n199 = local write "Export images"(w338) -> ()
        n200 = flat-sequence {
          tunnel: w338 -> [_]
          tunnel: w340 -> [w342]
          tunnel: [w342] -> w339
          frame #0 {
            n201 = local read "AVI File Path"() -> (w341:path)
            n202 = call "Export images from AVI file.vi"("AVI File Path"=w341) -> ()  [unwired: 11 in]
          }
        }
        n203 = call <vilib>:"Unset Busy.vi"("error in (no error)"=w339) -> ()  [unwired: 10 in, 1 out]
      }
    }
    n204 = local read "Stop (ind)"() -> (w336:bool)
  }
  n205 = while {
    shift-right: [w349] -> _
    shift-left: w19 -> [w348]
    tunnel: w30 -> [w347]
    shift-right: [w346] -> _
    shift-left: _ -> [w345]
    tunnel: [w344] -> w3
    tunnel: w4 -> [w343]
    tunnel: [w343] -> w5
    stop <- w350 stop-if-true
    # "EVENT HANDLING LOOP"
    n206 = event shown="[3] \"Scrollbar\": Value Change" {
      selector: _ -> [_ _ _ _ _ _ _ _ _ _ _ _ _ _ _ _ _ _]
      dyn-events: _ -> [_ _ _ _ _ _ _ _ _ _ _ _ _ _ _ _ _ _]
      timeout: 250 -> [_ _ _ _ _ _ _ _ _ _ _ _ _ _ _ _ _ _]
      tunnel: [w352 w358 _ _ _ _ _ _ _ _ _ _ _ _ _ _ _ w483] -> w350
      tunnel: [w356 w361 w372 w376 w385 w391 w399 w412 w426 w430 w437 w445 w450 w455 w459 w461 w478 w485] -> w349
      tunnel: w348 -> [w356 w361 w372 w378 w385 w391 w399 w414 w426 w430 w437 w445 w450 w455 w459 w463 w478 w485]
      tunnel: w347 -> [_ w359 _ w377 _ w392 _ w413 _ w429 _ _ _ w452 _ w467 _ w484]
      tunnel: [w355 w357 w373 w375 w384 w394 w398 w403 w422 w428 w433 FALSE FALSE w451 w458 w464 w477 w482] -> w346
      tunnel: w345 -> [w355 w357 w373 w375 w384 w394 w398 w403 w422 w428 _ w444 _ w451 w458 w464 w477 w482]
      tunnel: [w353 _ _ _ _ _ _ _ _ _ _ _ _ _ _ _ _ w481] -> w344
      tunnel: w343 -> [w354 _ _ _ _ _ _ _ _ _ _ _ _ _ _ _ _ w480]
      event Timeout {
        n207 = event-data() -> ()  [unwired: 1 in, 1 out]
        n208 = call "Bring Timelapse window to front.vi"() -> ()  [unwired: 12 in]
        n209 = global read "General Globals.vi" "Stop application"() -> (w352:bool)
        n210 = property class="VI"(reference=w354) -> ("FP.State"=w353:T22)  [unwired: 1 in, 2 out]
      }
      event Menu Selection (User) {
        n211 = event-data() -> ("ItemTag"=w360:string)  [unwired: 1 in]
        n212 = case shown="\"Close\"" w360 {
          tunnel: w359 -> [_ w362 _ _ w367 _ _ _]
          tunnel: [_ _ _ _ w366 _ _ _] -> w358
          frame Default {
          }
          frame "Load dataset" {
            n213 = call "Timelapse viewer-Event handler-Load dataset.vi"("queue"=w362) -> ()  [unwired: 11 in]
          }
          frame "Playback speed..." {
            n214 = call "Window-Playback speed entry.vi"() -> ("Frame rate set (fps)"=w363:dbl)  [unwired: 10 in, 1 out]
            n215 = local write "Frame rate set (fps)"(w363) -> ()
          }
          frame "Original speed (x1)" {
            n216 = flat-sequence {
              frame #0 {
                n217 = global write "gl_Time series viewer globals.vi" "Use manual FPS?"(FALSE ("Use manual FPS?")) -> ()
              }
              frame #1 {
                n218 = call "AVI playback timing control.vi"() -> ("Frame rate set OR original (fps)"=w365:dbl)  [unwired: 8 in, 3 out]
                n219 = local write "Frame rate set (fps)"(w365) -> ()
              }
            }
          }
          frame "Close" {
            n220 = call "Timelapse viewer-Event handler-Exit.vi"("Queue in"=w367) -> ("Exit"=w366:bool)  [unwired: 10 in]
            n221 = case shown="True" w366 {
              frame False {
              }
              frame True {
                n222 = local write "Stop"(TRUE ("Stop")) -> ()
              }
            }
          }
          frame "Export snippet" {
            "Export snippet" <- TRUE
          }
          frame "Export 8-bit video" {
            "Export vid" <- TRUE
          }
          frame "Export TIFF series" {
            "Export images" <- TRUE
          }
        }
      }
      event "Scrollbar", "Speed Graph": Shortcut Menu Selection (User) {
        n223 = event-data() -> ("ItemTag"=w374:string)  [unwired: 1 in]
        n224 = call "Timelapse viewer-Shortcut menu handler.vi"("ItemTag"=w374) -> ()  [unwired: 11 in]
      }
      event "Scrollbar": Value Change {
        n225 = event-data() -> ()  [unwired: 1 in, 1 out]
        n226 = call "Event case-Scrollbar value change.vi"("Tick count in"=w378, "Queue in"=w377) -> ("Tick count"=w376:u32)  [unwired: 8 in, 1 out]
      }
      event "Speed Graph": Shortcut Menu Activation? {
        n227 = event-data() -> ("MenuRef"=w381:refnum<k9>)  [unwired: 1 in]
        n228 = call "FGV_Speed graph behaviour-Main viewer.vi"("Function"=Get-Set-Clear_Control."Get") -> ("Speed graph behaviour"=w380:T23)  [unwired: 9 in, 1 out]
        n229 = case shown="\"Scrolling data\", Default" w380 {
          tunnel: [bool[] [FALSE, TRUE] bool[] [TRUE, FALSE]] -> w379
          frame "Scrolling data", Default {
          }
          frame "Scrolling cursor" {
          }
        }
        n230 = for {
          tunnel: string[] ["scrolling cursor", "scrolling data"] -> [w390] mode=indexing
          tunnel: w381 -> [w389]
          tunnel: w379 -> [w388] mode=indexing
          n231 = Set Menu Item Info(6:w388, 7:w390, 11:w389) -> ()  [unwired: 4 in, 2 out]
        }
        n232 = event-data() -> ()  [unwired: 2 in, 1 out]
      }
      event "Speed Graph": Cursor Move; "Speed Graph": Cursor Release {
        n233 = event-data() -> ("CursRef"=w393:refnum<vi>)  [unwired: 1 in]
        n234 = call "Event case-Speed graph cursor moved.vi"("queue in"=w392, "Cursor in"=w393) -> ()  [unwired: 9 in, 1 out]
      }
      event "Speed Graph": event type 3.0.x80000027 {
        n235 = event-data() -> ()  [unwired: 1 in, 1 out]
        n236 = call "FGV_Speed graph behaviour-Main viewer.vi"("Function"=Get-Set-Clear_Control."Get") -> ("Speed graph behaviour"=w396:T23)  [unwired: 9 in, 1 out]
        n237 = case shown="\"Scrolling data\", Default" w396 {
          tunnel: [TRUE FALSE] -> w395
          frame "Scrolling data", Default {
            # "Moving the speed data graph's cursor manually is \nprevented when the mode is \"Scrolling data\"."
          }
          frame "Scrolling cursor" {
            # "Moving the speed data graph's cursor manually is \nallowed when the mode is \"Scrolling cursor\"."
          }
        }
        n238 = event-data("Discard?"=w395) -> ()  [unwired: 1 in, 1 out]
      }
      event "Selection sliders": Value Change {
        # "Do not use the left cursor's change event"
        # "Sets the main slider to the value of the extraction cursor that was moved."
        n239 = event-data() -> ("OldVal"=w411:cluster{i32, i32}, "NewVal"=w404:cluster{i32, i32})  [unwired: 1 in]
        n240 = Not Equal?(x=w411, y=w404) -> (x != y?=w405:cluster{bool, bool})
        n241 = Unbundle(w405) -> (w402:bool)  [unwired: 1 out]
        n242 = Unbundle(w404) -> (w410:i32, w409:i32)
        n243 = Select(t=w409, s=w402, f=w410) -> (s? t:f=w406:i32)
        n244 = flat-sequence {
          tunnel: w413 -> [w417]
          tunnel: w414 -> [w418]
          tunnel: [w418] -> w408
          tunnel: [w417] -> w407
          tunnel: w406 -> [w416]
          tunnel: w402 -> [w415]
          tunnel: [w419] -> w412
          tunnel: w408 -> [w421]
          tunnel: w407 -> [w420]
          frame #0 {
            n245 = call "Sync scrollbars.vi"("Min cursor moved"=w415, "Scrollbar value"=w416) -> ()  [unwired: 9 in, 1 out]
          }
          frame #1 {
            n246 = call "Event case-Scrollbar value change.vi"("Tick count in"=w421, "Queue in"=w420) -> ("Tick count"=w419:u32)  [unwired: 8 in, 1 out]
          }
        }
      }
      event "Colour": Value Change {
        n247 = event-data() -> ()  [unwired: 1 in, 1 out]
        n248 = call "Set image colour.vi"("Left Image Palette"="Colour") -> ("Color Palette"=w423:cluster{"Red":u8, "Green":u8, "Blue":u8}[], "Palette Type"=w424:u32)  [unwired: 9 in]
        n249 = property on="Image" class="ImageControl"("Palette Type"=w424, "User Palette"=w423) -> ()  [unwired: 2 in, 2 out]
      }
      event "AVI File Path": Value Change {
        w427 = TRUE ("Stop")
        n250 = event-data() -> ()  [unwired: 1 in, 1 out]
        n251 = local write "Stop"(w427) -> ()
        n252 = flat-sequence {
          tunnel: w429 -> [w432]
          tunnel: w427 -> [_]
          frame #0 {
            n253 = Enqueue Element At Opposite End(queue=w432, element=Speed_Viewer_States_enum."Initialise") -> ()  [unwired: 2 in, 3 out]
          }
        }
      }
      event "Cams.Vid 1", "Cams.Vid 2", "Cams.Vid 3", "Cams.Vid 4": Mouse Down {
        # "http://zone.ni.com/reference/en-XX/help/371361K-01/lvhowto/drag_and_drop_programmatic_prepare/"
        # "Detects and registers when the mouse is clicked \nwithin the boundaries of a CamVid display. This allows to generate a \"Drag leave\" event for those displays (in a separate event case / Mouse leave case).\nThis is necessary because the Drag-Leave event does not work for this type of control."
        n254 = event-data() -> ("Button"=w434:u16, "Mods.Double Click"=w436:bool, "CtlRef"=w435:refnum<vi>)  [unwired: 1 in]
        n255 = case shown="True" w436 {
          tunnel: w434 -> [_ w439]
          tunnel: w435 -> [_ w441]
          frame False {
          }
          frame True {
            n256 = property class="ImageControl"(reference=w441) -> ("Label.Text"=w440:string)  [unwired: 1 in, 2 out]
            n257 = call "Open expanded image window.vi"("Button"=w439, "Image name"=w440) -> ()  [unwired: 10 in]
          }
        }
        n258 = case shown="1" w434 {
          tunnel: [_ TRUE] -> w433
          frame 0, Default {
          }
          frame 1 {
          }
        }
      }
      event "Cams.Vid 1", "Cams.Vid 2", "Cams.Vid 3", "Cams.Vid 4": Mouse Leave {
        n259 = event-data() -> ("CtlRef"=w442:refnum<vi>)  [unwired: 1 in]
        n260 = case shown="False" w444 {
          tunnel: w442 -> [_ w448]
          frame False {
          }
          frame True {
            n261 = property class="ImageControl"(reference=w448) -> ("Label.Text"=w446:string)  [unwired: 1 in, 2 out]
            n262 = call "Open expanded image window.vi"("Button"=u16 0, "Image name"=w446) -> ()  [unwired: 10 in]
          }
        }
      }
      event Mouse Up {
        n263 = event-data() -> ()  [unwired: 1 in, 1 out]
      }
      event "Back": Value Change {
        n264 = event-data() -> ()  [unwired: 1 in, 1 out]
        n265 = Enqueue Element At Opposite End(queue=w452, element=Speed_Viewer_States_enum."Back to start") -> ()  [unwired: 2 in, 3 out]
        n266 = local write "Stop"(TRUE ("Stop")) -> ()
      }
      event Value Change {
        n267 = event-data() -> ()  [unwired: 1 in, 1 out]
        n268 = global write "gl_Time series viewer globals.vi" "Intensity"("Intensity") -> ()
        n269 = call "16-bit display mapping.vi"() -> ("16-bit Display Mapping"=w457:T15)  [unwired: 10 in, 1 out]
        n270 = property on="Image" class="ImageControl"("16-bit Display Mapping"=w457) -> ()  [unwired: 2 in, 2 out]
      }
      event "Play": Value Change {
        n271 = event-data() -> ()  [unwired: 1 in, 1 out]
        n272 = flat-sequence {
          tunnel: w467 -> [w471]
          tunnel: [w471] -> w466
          tunnel: w463 -> [w468]
          tunnel: [w468] -> w462
          tunnel: w466 -> [w473]
          tunnel: [w473] -> w465
          tunnel: w462 -> [w472]
          tunnel: [w472] -> w460
          tunnel: w465 -> [w475]
          tunnel: [w474] -> w461
          tunnel: w460 -> [w474]
          frame #0 {
            n273 = local write "Stop"(FALSE ("Stop")) -> ()
            n274 = call "Set Play-Stop buttons.vi"("Function"=Select_Play-Stop_button_to_show."Show Stop button") -> ()  [unwired: 10 in, 1 out]
          }
          frame #1 {
            n275 = call "Set scrollbar at start.vi"("Queue in"=w473) -> ()  [unwired: 10 in, 1 out]
          }
          frame #2 {
            n276 = Enqueue Element(queue=w475, element=Speed_Viewer_States_enum."Playback" ("States")) -> ()  [unwired: 2 in, 3 out]
          }
        }
      }
      event "Stop": Value Change {
        n277 = event-data() -> ()  [unwired: 1 in, 1 out]
      }
      event Panel Close? {
        # "The panel close is always discarded here because it is closed conditionally in the yellow \"Save Windows Bounds\" vi."
        n278 = event-data() -> ()  [unwired: 1 in, 1 out]
        n279 = call "Timelapse viewer-Event handler-Exit.vi"("Queue in"=w484) -> ("Exit"=w483:bool)  [unwired: 10 in]
        n280 = case shown="True" w483 {
          frame False {
          }
          frame True {
            n281 = local write "Stop"(TRUE ("Stop")) -> ()
            n282 = global write "gl_Time series viewer globals.vi" "Close larger image windows"(TRUE ("Close larger image window")) -> ()
          }
        }
        n283 = property class="VI"(reference=w480) -> ("FP.State"=w481:T22)  [unwired: 1 in, 2 out]
        n284 = event-data("Discard?"=TRUE) -> ()  [unwired: 1 in, 1 out]
      }
    }
  }
  n285 = disable-structure shown="Disabled" {
    frame Disabled {
      # "AVI1 VIs"
      n286 = call "IMAQ AVI Create"() -> ()  [unwired: 10 in, 2 out]
      n287 = call "IMAQ AVI Open"() -> ()  [unwired: 10 in, 2 out]
      n288 = call "IMAQ AVI Read Frame"() -> ()  [unwired: 8 in, 4 out]
      n289 = call "IMAQ AVI Write Frame"() -> ()  [unwired: 10 in, 2 out]
      n290 = call "IMAQ AVI Get Info"() -> ()  [unwired: 7 in, 5 out]
      n291 = call "IMAQ AVI Close"() -> ()  [unwired: 11 in, 1 out]
    }
    frame Enabled {
    }
  }
  n292 = call "AVI-Viewer cleanup.vi"("error in (no error)"=w27, "RGB image ref"=w17, "I16 image ref"=w31) -> ("error out"=w2:errorcluster)  [unwired: 8 in]
  n293 = flat-sequence {
    tunnel: w7 -> [w491]
    tunnel: w5 -> [w489]
    tunnel: w3 -> [w488]
    tunnel: w2 -> [_]
    frame #0 {
      n294 = call "Save_Windows_Bounds.vi"("FP.State"=w488, "Window Name (i.e. Key)"=w491, "Front Panel Window:Open"=FALSE, "Window VI's Ref"=w489) -> ()  [unwired: 7 in, 1 out]
    }
  }
